vi "TurretSystem.vi"() -> ()   [LabVIEW 2025]
panel:
  out "TurretLauncher/TurretPos":dbl caption="Pos Deg" format="%12.1f"
  out "TurretLauncher/OnTarget":bool caption="On Target"
  out "TurretLauncher/TurretMotorOut":dbl caption="Motor Output" format="%11.2f"
  out "TurretLauncher/TurretPosDmd":dbl caption="Pos Dmd Deg" format="%12.1f"
  out "TurretLauncher/CWLimit":bool caption="CW Limit"
  out "TurretLauncher/CCWLimit":bool caption="CCW Limit"
  # "TURRET"
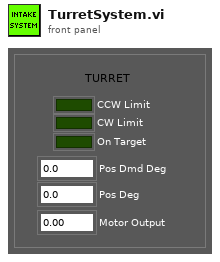
[diagram p1: front panel]
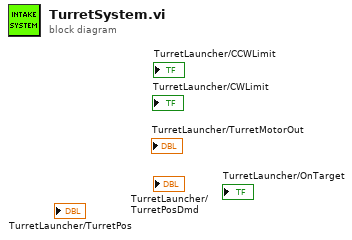
[diagram p0: block diagram]
diagram:
